vi "CSM - Flood of Events Handler Side Loop.vi"() -> ()   [LabVIEW 2017, in "CSM-QuickDrops.lvlib"]
doc: "User Event Structure loop template for DQMH-style CSM modules. This VI is primarily used for handling scenarios where user interface operations are very complex and require combined logic to complete collaborative work.\n\n<b>Reference Example</b>: `[CSM-Example]\\4. Advance Examples\\CSMLS - Continuous Loop in CSM Example.vi`."
uses:
  CSM-QuickDrops.lvlib
  _Polymophic/CSM - Filter Duplicated Lines.vi
  Communicable State Machine.lvlib
panel:
  in  "Slide":dbl(slide) scale=0.0..10.0
  in  "CSM Module":string
  # "Flood of Events:\n\nPanel/Pane Size Event\nSlide/Knob... User Event by dragging\nNumeric Control Value Change Event by Arraw Button"
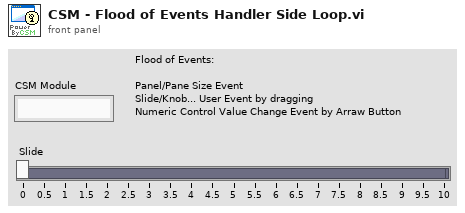
[diagram p1: front panel]
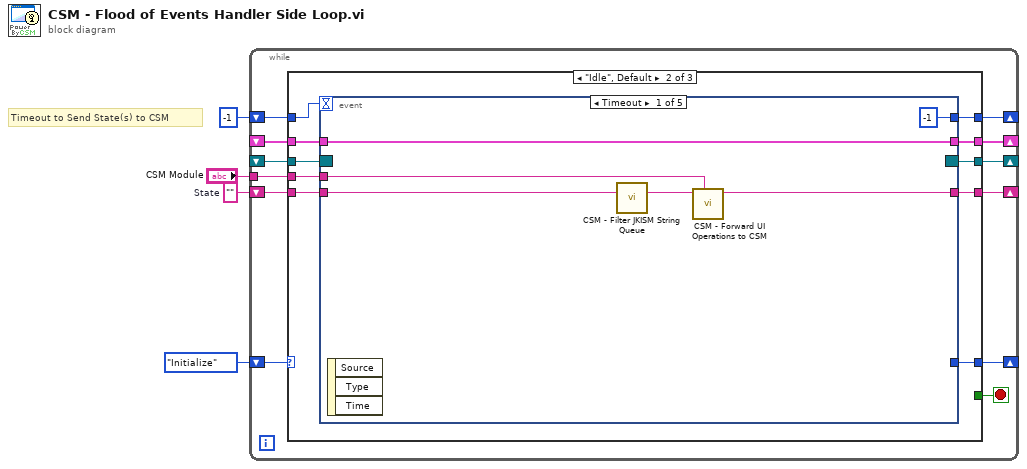
[diagram p0: block diagram]
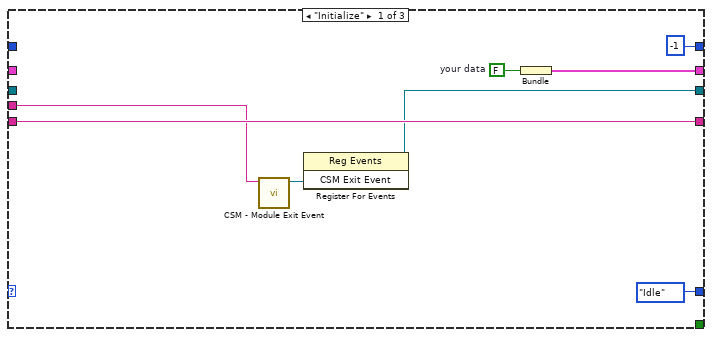
[diagram p2: hidden frame]
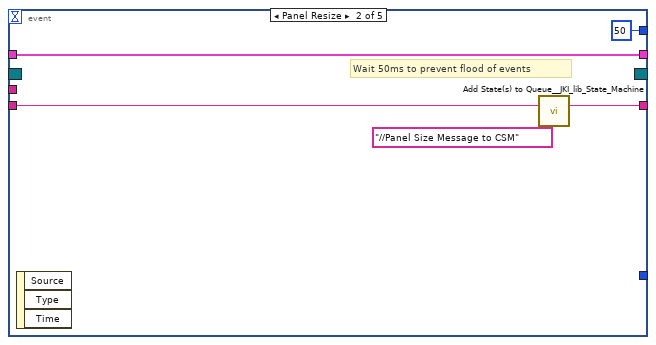
[diagram p3: hidden frame]
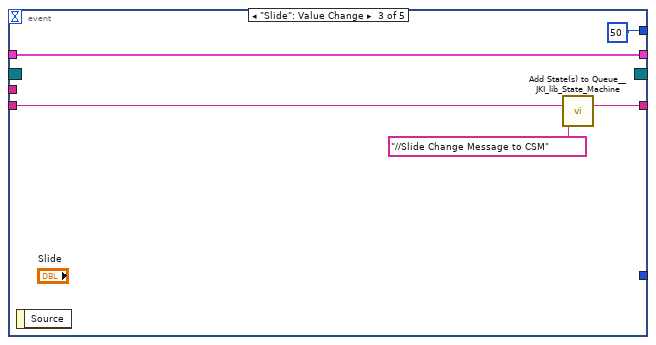
[diagram p4: hidden frame]
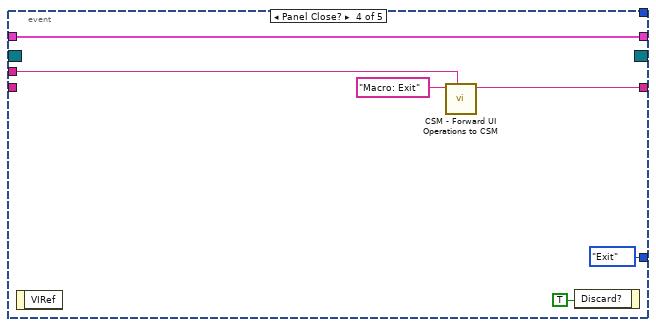
[diagram p5: hidden frame]
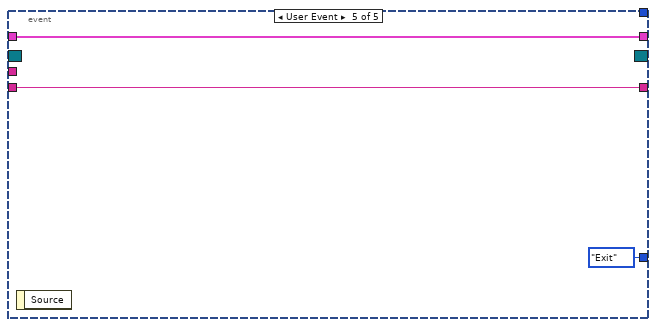
[diagram p6: hidden frame]
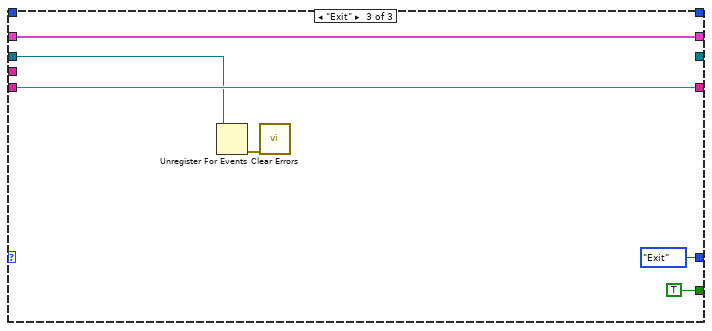
[diagram p7: hidden frame]
diagram:
  w3 = ""  # State
  # "Timeout to Send State(s) to CSM"
  n1 = while {
    shift-right: [w15] -> _
    shift-left: enum16{"Idle", "Initialize", "Exit"}."Initialize" -> [w16]
    tunnel: "CSM Module" -> [w13]
    shift-right: [w11] -> _
    shift-left: w3 -> [w12]
    shift-right: [w9] -> _
    shift-left: -1 -> [w10]
    shift-right: [w8] -> _
    shift-left: _ -> [w7]
    shift-right: [w6] -> _
    shift-left: _ -> [w5]
    stop <- w14 stop-if-true
    n2 = case shown="\"Idle\", Default" w16 {
      tunnel: [enum16{"Idle", "Initialize", "Exit"}."Idle" w34 enum16{"Idle", "Initialize", "Exit"}."Exit"] -> w15
      tunnel: [_ _ TRUE] -> w14
      tunnel: w13 -> [w20 w33 _]
      tunnel: w12 -> [w23 w31 w63]
      tunnel: [w23 w32 w63] -> w11
      tunnel: w10 -> [_ w29 _]
      tunnel: [-1 w30 _] -> w9
      tunnel: [w19 w27 _] -> w8
      tunnel: w7 -> [_ w28 w62]
      tunnel: [w17 w25 w60] -> w6
      tunnel: w5 -> [_ w26 w60]
      frame "Initialize" {
        w18 = FALSE  # your data
        n3 = call "CSM - Module Exit Event.vi"("Name (\"\" to Use UUID) In"=w20) -> ("CSM Exit Event"=w21:refnum<user-event>)  [unwired: 8 in, 2 out]
        n4 = register-events(w21) -> (reference out=w19:refnum<event-registration>)  [unwired: 2 in, 1 out]
        n5 = Bundle("your data"=w18) -> (w17:cluster{"your data":bool})  [unwired: 1 in]
      }
      frame "Idle", Default {
        n6 = event shown="[0] Timeout" {
          selector: w28 -> [_ _ _ _ _]
          dyn-events: [_ _ _ _ _] -> w27
          timeout: w29 -> [_ _ _ _ _]
          tunnel: [_ _ _ enum16{"Idle", "Initialize", "Exit"}."Exit" enum16{"Idle", "Initialize", "Exit"}."Exit"] -> w34
          tunnel: w33 -> [w38 _ _ w53 _]
          tunnel: w31 -> [w36 w45 w50 _ w59]
          tunnel: [w39 w44 w49 w52 w59] -> w32
          tunnel: [-1 50 50 _ _] -> w30
          tunnel: w26 -> [w37 w41 w46 w51 w57]
          tunnel: [w37 w41 w46 w51 w57] -> w25
          event Timeout {
            n7 = event-data() -> ()  [unwired: 1 in, 3 out]
            n8 = call-poly "CSM - Filter JKISM String Queue.vi"("States In"=w36) -> ("States Out"=w35:string)  [unwired: 14 in]
            n9 = call "CSM - Forward UI Operations to CSM.vi"("Name (\"\" to Use UUID)"=w38, "State(s) In (\"\")"=w35) -> ("States Out"=w39:string)  [unwired: 8 in, 1 out]
          }
          event Panel Resize {
            # "Wait 50ms to prevent flood of events"
            n10 = event-data() -> ()  [unwired: 1 in, 3 out]
            n11 = call <vilib>:"Add State(s) to Queue__JKI_lib_State_Machine.vi"("State(s) in (\"\")"=w45, "State(s) at Back (\"\")"="//Panel Size Message to CSM" ("State(s) at Back (\"\")")) -> ("States Out"=w44:string)  [unwired: 13 in]
          }
          event "Slide": Value Change {
            n12 = event-data() -> ()  [unwired: 1 in, 1 out]
            n13 = call <vilib>:"Add State(s) to Queue__JKI_lib_State_Machine.vi"("State(s) in (\"\")"=w50, "State(s) at Back (\"\")"="//Slide Change Message to CSM" ("State(s) at Back (\"\")")) -> ("States Out"=w49:string)  [unwired: 13 in]
          }
          event Panel Close? {
            n14 = event-data() -> ()  [unwired: 1 in, 1 out]
            n15 = call "CSM - Forward UI Operations to CSM.vi"("Name (\"\" to Use UUID)"=w53, "State(s) In (\"\")"="Macro: Exit" ("State")) -> ("States Out"=w52:string)  [unwired: 8 in, 1 out]
            n16 = event-data("Discard?"=TRUE) -> ()  [unwired: 1 in, 1 out]
          }
          event User Event {
            n17 = event-data() -> ()  [unwired: 1 in, 1 out]
          }
        }
      }
      frame "Exit" {
        n18 = Unregister For Events(event registration refnum=w62) -> (error out=w61:errorcluster)  [unwired: 1 in]
        n19 = call <vilib>:"Clear Errors.vi"("error in (no error)"=w61) -> ()  [unwired: 5 in, 2 out]
      }
    }
  }
